vi "Parse path.vi"(8 "error in":errorcluster, 10 "Paths?":variant) -> (0 "error out":errorcluster, 2 "Paths":string[](array[string]))   [LabVIEW 2013, in "Data.PGSQL.lvclass"]
uses:
  Data.PGSQL.lvclass
  Typedefs/Errors--enum.ctl
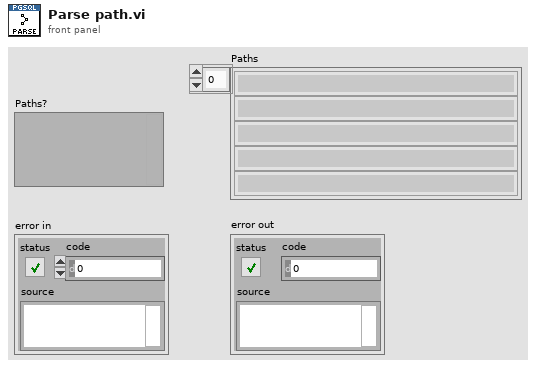
[diagram p1: front panel]
types:
  T1 = enum8{"<Null>", "I8", "I16", "I32", "I64", "U8", "U16", "U32", "U64", "SGL", "DBL", "EXT", "CSG", "CDB", "CXT", "0x0F", "0x10", "0x11", "0x12", "0x13", "0x14", "Enum U8", "Enum U16", "Enum U32", "Enum U64", "SGL PQ", "DBL PQ", "EXT PQ", "CSG PQ", "CDB PQ", "CXT PQ", "0x1F", "0x20", "Boolean", "0x22", "0x23", "0x24", "0x25", "0x26", "0x27", "0x28", "0x29", "0x2A", "0x2B", "0x2C", "0x2D", "0x2E", "0x2F", "String", "0x31", "Path", "Pict", "0x34", "0x35", "0x36", "DAQ", "0x38", "0x39", "0x3A", "0x3B", "0x3C", "0x3D", "0x3E", "0x3F", "Array", "0x41", "0x42", "0x43", "0x44", "0x45", "0x46", "0x47", "0x48", "0x49", "0x4A", "0x4B", "0x4C", "0x4D", "0x4E", "0x4F", "Cluster", "0x51", "0x52", "Variant", "Waveform", "0x55", "0x56", "0x57", "0x58", "0x59", "0x5A", "0x5B", "0x5C", "0x5D", "0x5E", "0x5F", "0x60", "0x61", "0x62", "0x63", "0x64", "0x65", "0x66", "0x67", "0x68", "0x69", "0x6A", "0x6B", "0x6C", "0x6D", "0x6E", "0x6F", "Refnum"}
  T2 = typedef "Data.PGSQL.lvclass/Errors--enum.ctl" = enum16{"0: None", "5005: Path Type Not Supported", "5006: Number of Variables", "5008: Cannot write two data points", "5030: Start and End Times Identical", "5031: Input is not wholly", "5033: Bad path or paths", "5040: Invalid Instrument Name", "5050: Column can only hold string", "5051 Column can only hold bool", "5052: Column can only hold double", "5053: Column can only hold int"}
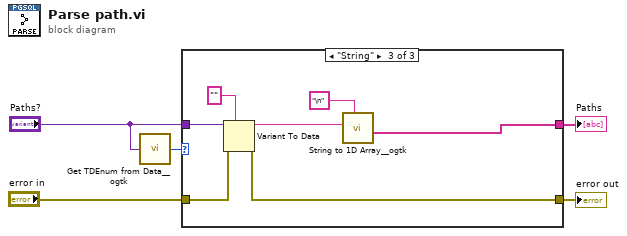
[diagram p0: block diagram]
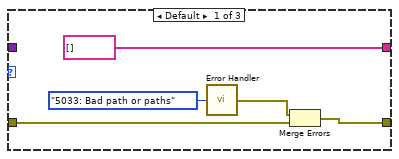
[diagram p2: hidden frame]
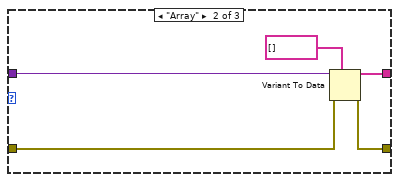
[diagram p3: hidden frame]
diagram:
  n1 = call "Get TDEnum from Data__ogtk.vi"("Data"="Paths?") -> ("Type Descriptor Enumeration"=w3:T1)  [unwired: 4 in]
  n2 = case shown="\"String\"" w3 {
    tunnel: "Paths?" -> [_ w15 w21]
    tunnel: [string[] [] w13 w19] -> w5
    tunnel: "error in" -> [w9 w12 w17]
    tunnel: [w8 w11 w16] -> w4
    frame Default {
      n3 = call "Error Handler.vi"("Error code"=Errors--enum."5033: Bad path or paths") -> ("error out"=w7:errorcluster)
      n4 = Merge Errors(w7, w9) -> (w8:errorcluster)
    }
    frame "Array" {
      n5 = Variant To Data(error in=w12, type=string[] [], Variant=w15) -> (data=w13:string[], error out=w11:errorcluster)
    }
    frame "String" {
      n6 = Variant To Data(error in=w17, type="", Variant=w21) -> (data=w20:string, error out=w16:errorcluster)
      n7 = call <userlib>:"String to 1D Array__ogtk.vi"("delimiter (Tab)"="\n", "string"=w20) -> ("Array of Strings"=w19:string[])  [unwired: 9 in]
    }
  }
  "Paths" <- w5
  "error out" <- w4
